vi "niScope Send Software Trigger Edge.vi"(0 "instrument handle":refnum<k15>, 5 "which trigger":u16(ring) items=["StartTrigger", "ArmReferenceTrigger", "ReferenceTrigger", "AdvanceTrigger"], 11 "error in":errorcluster) -> (4 "instrument handle out":refnum<k15>, 15 "error out":errorcluster)   [LabVIEW 2011]
doc: "Sends the selected trigger to the digitizer. If you called niScope Configure Trigger Software, call this VI when you want the reference trigger to occur. You can also call this VI to override a misused edge, digital, or hysteresis reference trigger. If you have configured an Acquisition Arm Source, an Arm Reference Trigger Source, or an Advance Trigger Source, call this VI when you want to send the corresponding trigger to the digitizer."
uses:
  niScope_32.dll
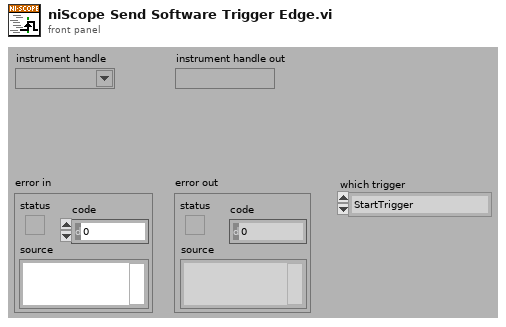
[diagram p1: front panel]
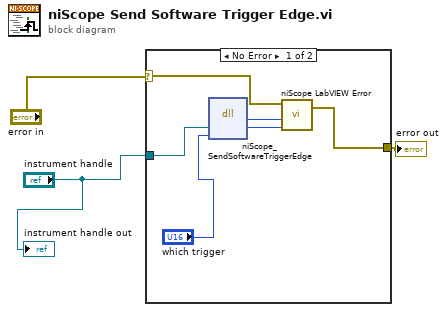
[diagram p0: block diagram]
diagram:
  n1 = case shown="No Error" "error in" {
    selector: "error in" -> [w4 w10]
    tunnel: [w8 w10] -> w3
    tunnel: "instrument handle" -> [w9 _]
    frame No Error {
      n2 = dll-call lib="niScope_*.*" fn="niScope_SendSoftwareTriggerEdge"("instrument handle"=w9, "whichTrigger"="which trigger") -> ("status"=w7:i32, "instrument handle"=w6:u32)  [unwired: 4 in, 2 out]
      n3 = call <instrlib>:"niScope LabVIEW Error.vi"("instrument handle"=w6, "niScope error code (0)"=w7, "error in (no error)"=w4) -> ("error out"=w8:errorcluster)  [unwired: 2 in]
    }
    frame Error {
    }
  }
  "error out" <- w3
  "instrument handle out" <- "instrument handle"
